vi "Init.vi"(0 "DevControl 输入":refnum<class "DevControl.lvclass"> caption="DNL_LabVIEW Object in", 5 "控制端口":refnum<visa-resource-name>, 7 "波特率":u32, 9 "ReadDelay":u32, 11 "error in (no error)":errorcluster caption="错误输入（无错误）", 12 "Retry":i32) -> (4 "DevControl 输出":refnum<class "DevControl.lvclass"> caption="DNL_LabVIEW Object out", 15 "error out":errorcluster caption="错误输出")   [LabVIEW 2012, in "DevControl.lvclass"]
uses:
  DevControl.lvclass
  Libs/Serial/Serial.lvclass
  DevControl.lvclass/DevControl.ctl
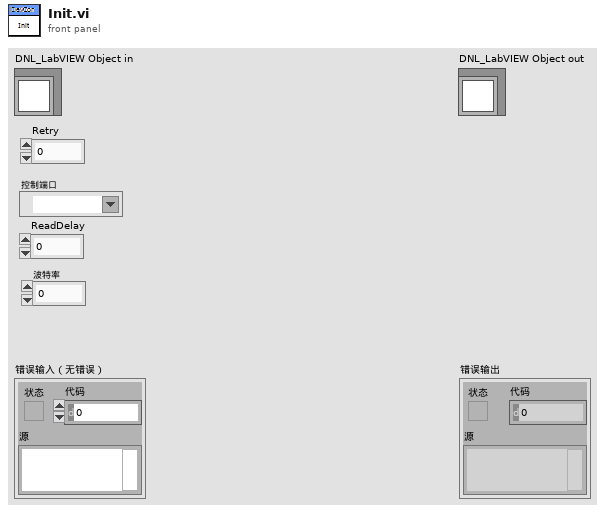
[diagram p1: front panel]
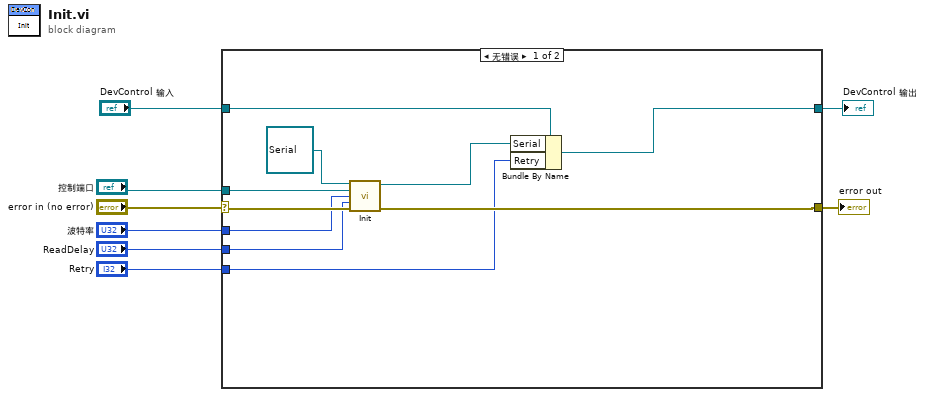
[diagram p0: block diagram]
diagram:
  n1 = case shown="无错误" "error in (no error)" {
    selector: "error in (no error)" -> [w18 w20]
    tunnel: [w17 w20] -> w7
    tunnel: [w15 w19] -> w5
    tunnel: "DevControl 输入" -> [w16 w19]
    tunnel: "控制端口" -> [w14 _]
    tunnel: "波特率" -> [w13 _]
    tunnel: "ReadDelay" -> [w12 _]
    tunnel: "Retry" -> [w9 _]
    frame No Error {
      n2 = call-dynamic "Init.vi"("Serial 输入"=refnum<class "Serial.lvclass"> refnum, "控制端口"=w14, "波特率"=w13, "ReadDelay"=w12, "error in (no error)"=w18) -> ("Serial 输出"=w11:refnum<class "Serial.lvclass">, "error out"=w17:errorcluster)  [unwired: 9 in]
      n3 = Bundle By Name(cluster=w16, "Serial"=w11, "Retry"=w9) -> (w15:refnum<class "DevControl.lvclass">)
    }
    frame Error {
    }
  }
  "error out" <- w7
  "DevControl 输出" <- w5
